vi "Display_data_dates.vi"(1 "String":string) -> (0 "resulting string":string)   [LabVIEW 2010]
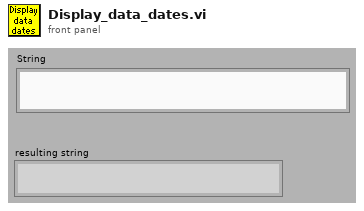
[diagram p1: front panel]
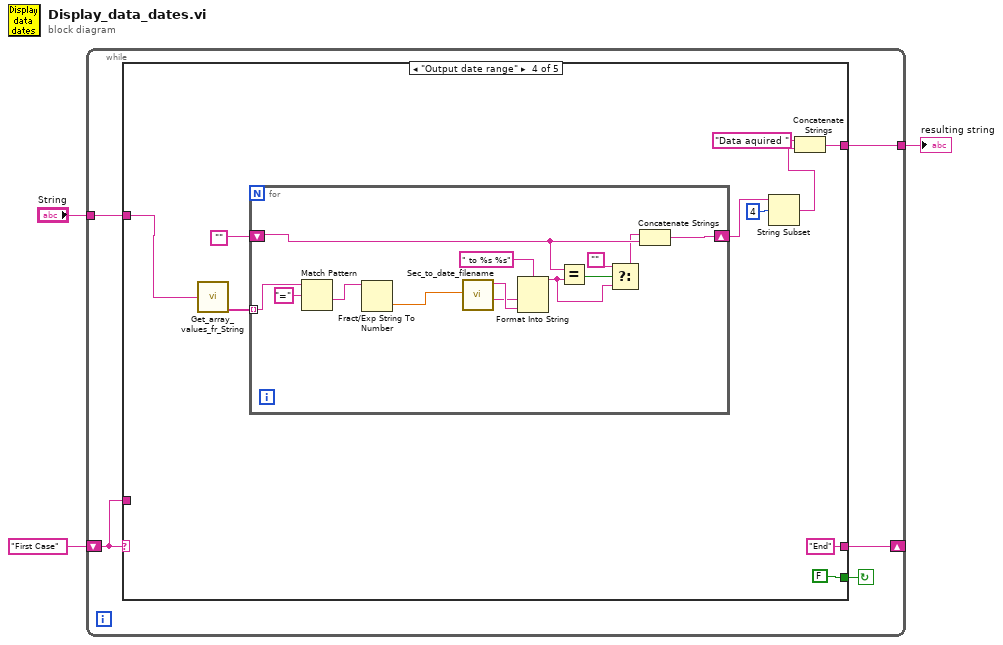
[diagram p0: block diagram]
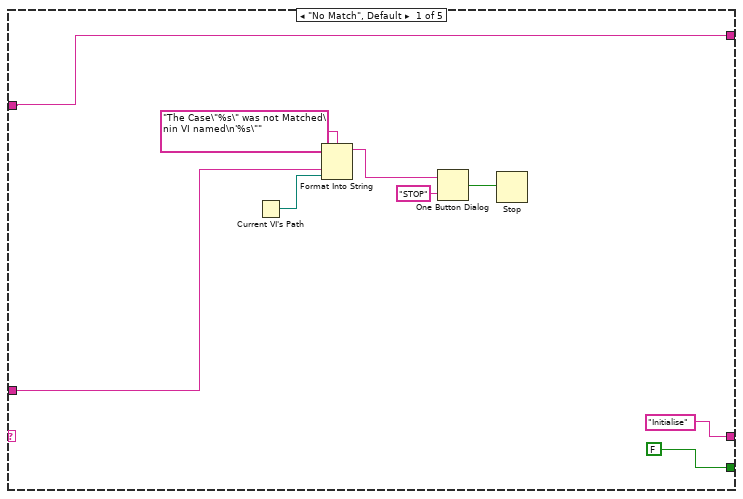
[diagram p2: hidden frame]
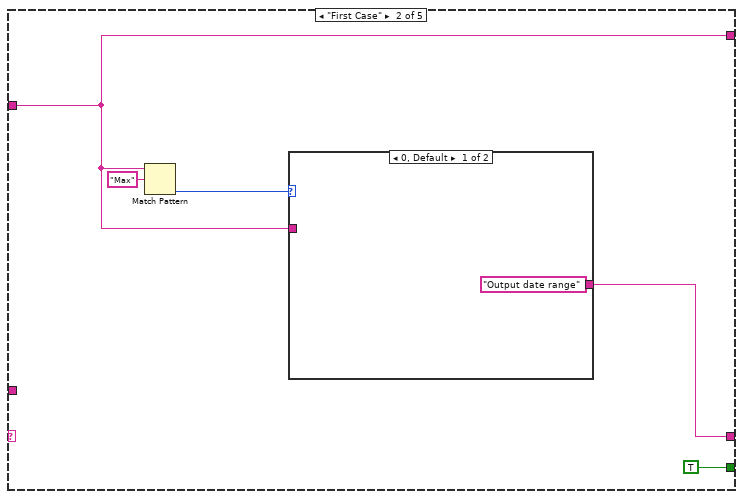
[diagram p3: hidden frame]
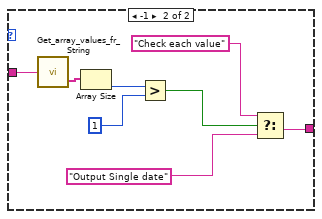
[diagram p4: hidden frame]
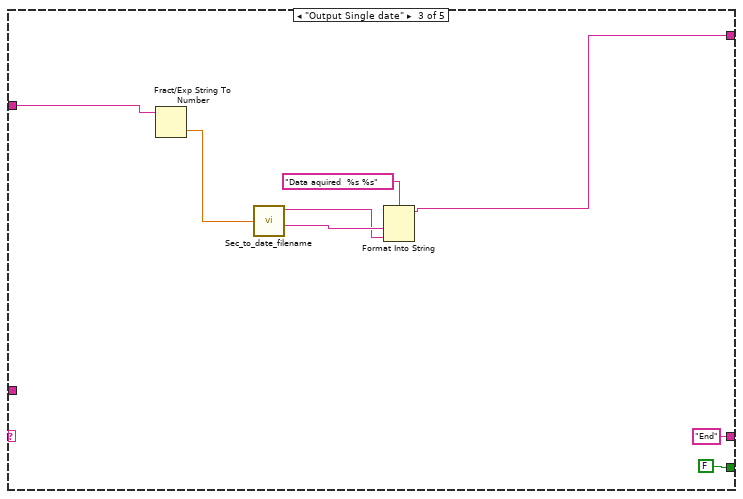
[diagram p5: hidden frame]
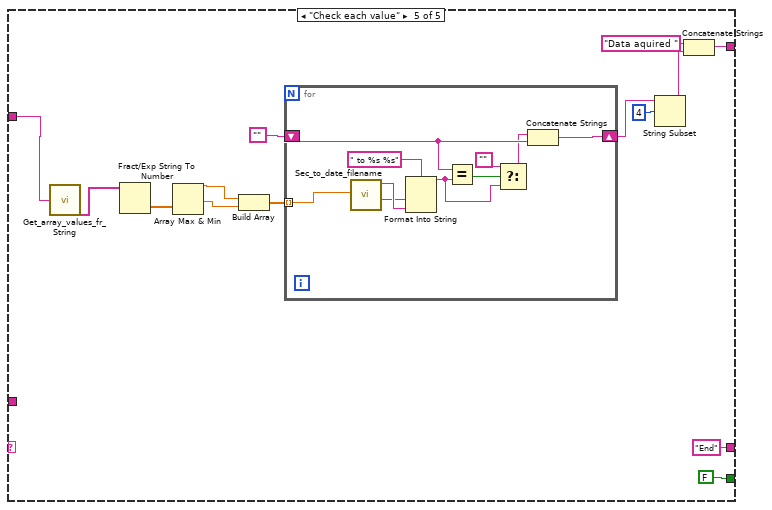
[diagram p6: hidden frame]
diagram:
  n1 = while {
    shift-left: "First Case" -> [w6]
    shift-right: [w7] -> _
    tunnel: "String" -> [w5]
    tunnel: [w4] -> w1
    stop <- w8 continue-if-true
    n2 = case shown="\"Output date range\"" w6 {
      tunnel: [FALSE TRUE FALSE FALSE FALSE] -> w8
      tunnel: ["Initialise" w19 "End" "End" "End"] -> w7
      tunnel: w6 -> [w12 _ _ _ _]
      tunnel: w5 -> [w9 w18 w34 w48 w75]
      tunnel: [w9 w18 w33 w40 w64] -> w4
      frame "No Match", Default {
        n3 = Current VI's Path() -> (path=w11:path)
        n4 = Format Into String(format string="The Case\"%s\" was not Matched\nin VI named\n'%s\"" ("Format String"), w12, w11) -> (resulting string=w15:string)  [unwired: 2 in, 1 out]
        n5 = One Button Dialog(message=w15, button name ("OK")="STOP") -> (true=w13:bool)
        n6 = Stop(stop? (T)=w13) -> ()
      }
      frame "First Case" {
        n7 = Match Pattern(string=w18, regular expression="Max") -> (offset past match=w20:i32)  [unwired: 4 out]
        n8 = case shown="0, Default" w20 {
          tunnel: ["Output date range" w25] -> w19
          tunnel: w18 -> [_ w31]
          frame 0, Default {
          }
          frame -1 {
            n9 = call "Get_array_values_fr_String.vi"("String Value"=w31) -> ("String array"=w30:string[])  [unwired: 1 out]
            n10 = Array Size(array=w30) -> (size(s)=w29:i32)
            n11 = Greater?(x=w29, y=1) -> (0:w27:bool)
            n12 = Select(t="Check each value", s=w27, f="Output Single date") -> (s? t:f=w25:string)
          }
        }
      }
      frame "Output Single date" {
        n13 = Fract/Exp String To Number(string=w34) -> (number=w38:dbl)  [unwired: 4 out]
        n14 = call "Sec_to_date_filename.vi"("seconds"=w38) -> ("Year"=w36:string, "Day"=w37:string)  [unwired: 2 out]
        n15 = Format Into String(format string="Data aquired  %s %s", w37, w36) -> (resulting string=w33:string)  [unwired: 2 in, 1 out]
      }
      frame "Output date range" {
        n16 = call "Get_array_values_fr_String.vi"("String Value"=w48) -> ("String array"=w47:string[])  [unwired: 1 out]
        n17 = for {
          tunnel: w47 -> [w61] mode=indexing
          shift-right: [w55] -> w43
          shift-left: "" -> [w54]
          n18 = Match Pattern(string=w61, regular expression="=") -> (after substring=w60:string)  [unwired: 4 out]
          n19 = Fract/Exp String To Number(string=w60) -> (number=w56:dbl)  [unwired: 4 out]
          n20 = call "Sec_to_date_filename.vi"("seconds"=w56) -> ("Year"=w58:string, "Day"=w57:string)  [unwired: 2 out]
          n21 = Format Into String(format string=" to %s %s", w57, w58) -> (resulting string=w52:string)  [unwired: 2 in, 1 out]
          n22 = Equal?(x=w54, y=w52) -> (x = y?=w53:bool)
          n23 = Select(t="", s=w53, f=w52) -> (s? t:f=w50:string)
          n24 = Concatenate Strings(w50, w54) -> (w55:string)
        }
        n25 = String Subset(string=w43, offset (0)=4) -> (substring=w41:string)  [unwired: 1 out]
        n26 = Concatenate Strings("Data aquired " ("string"), w41) -> (w40:string)
      }
      frame "Check each value" {
        n27 = call "Get_array_values_fr_String.vi"("String Value"=w75) -> ("String array"=w70:string[])  [unwired: 1 out]
        n28 = Fract/Exp String To Number(string=w70) -> (number=w69:dbl[])  [unwired: 4 out]
        n29 = Array Max & Min(array=w69) -> (max value=w68:dbl, min value=w67:dbl)  [unwired: 2 out]
        n30 = Build Array(w68, w67) -> (w66:dbl[])
        n31 = for {
          shift-right: [w83] -> w71
          shift-left: "" -> [w82]
          tunnel: w66 -> [w77] mode=indexing
          n32 = call "Sec_to_date_filename.vi"("seconds"=w77) -> ("Year"=w85:string, "Day"=w84:string)  [unwired: 2 out]
          n33 = Format Into String(format string=" to %s %s", w84, w85) -> (resulting string=w80:string)  [unwired: 2 in, 1 out]
          n34 = Equal?(x=w82, y=w80) -> (x = y?=w81:bool)
          n35 = Select(t="", s=w81, f=w80) -> (s? t:f=w78:string)
          n36 = Concatenate Strings(w78, w82) -> (w83:string)
        }
        n37 = String Subset(string=w71, offset (0)=4) -> (substring=w65:string)  [unwired: 1 out]
        n38 = Concatenate Strings("Data aquired " ("string"), w65) -> (w64:string)
      }
    }
  }
  "resulting string" <- w1
